vi "SENS_CORR_COLL_SAVE.vi"(0 "VISA IN":refnum<visa-resource-name>, 5 "error in":errorcluster, 7 "Channel":i32) -> (14 "VISA Out":refnum<visa-resource-name>, 19 "error out":errorcluster)   [LabVIEW 2018, in "PNA-X.lvlib"]
doc: "SENSe<cnum>:CORRection:COLLect:SAVE \n1630\n\n(Write-only) For UNGUIDED calibrations ONLY. This command does the following: \ncalculates the error terms using the selected :METHod, \napplies the error terms to the selected measurement (turns error correction ON.) \nsaves the calibration error-terms to the channels Cal Register or a User Cal Set. \nThe Cal Register or User Cal Set is determined by the setting of the \nSENS:CORR:PREFerence:CSET:SAVE command. \nDo NOT use this command during an ECAL. When performing an ECAL calibration using \nSENS:CORR:COLL:ACQuire, this SAVE operation is performed automatically before the \ncompletion of a successful ACQuire. \nBefore using this command you must select a measurement using CALC:PAR:SEL. You can select \none measurement for each channel. \nParameters \n<cnum> Any existing channel number. If unspecified, value is set to 1 \nExamples SENS:CORR:COLL:SAVE \nsense2:correction:collect:save \nQuery Syntax Not applicable \nDefault Not applicable \nSENSe:CORRection:IMPedance:INPut:MAGNitude <num> \n(Read-Write) Sets and returns the system impedance value for the analyzer. \nParameters \n<num> System Impedance value in ohms. Choose any number between 0 and 1000 \nohms. \nExamples SENS:CORR:IMP:INP:MAGN 75 \nsense:correction:impedance:input:magnitude 50.5 \nQuery Syntax SENSe:CORRection:IMPedance: \nINPut:MAGNitude? \nReturn Type Numeric \nDefault 50 \n1631"
uses:
  PNA-X.lvlib
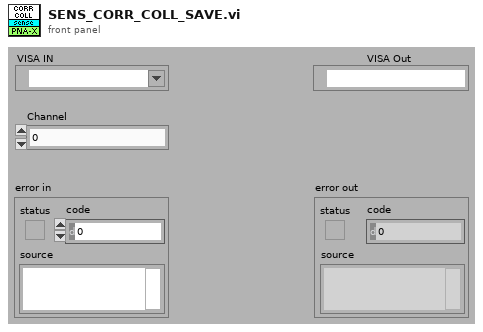
[diagram p1: front panel]
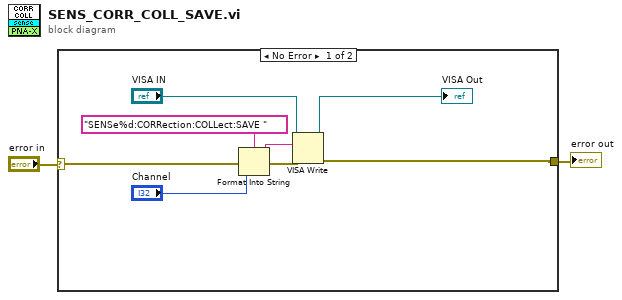
[diagram p0: block diagram]
diagram:
  n1 = case shown="No Error" "error in" {
    selector: "error in" -> [w10 w11]
    tunnel: [w5 w11] -> w1
    frame No Error {
      n2 = Format Into String(format string="SENSe%d:CORRection:COLLect:SAVE " ("Cmdline"), error in=w10, "Channel") -> (resulting string=w8:string, error out=w9:errorcluster)  [unwired: 1 in]
      n3 = VISA Write(VISA resource name="VISA IN", write buffer=w8, error in (no error)=w9) -> (VISA resource name out=→"VISA Out":refnum<visa-resource-name>, error out=w5:errorcluster)  [unwired: 1 out]
    }
    frame Error {
    }
  }
  "error out" <- w1
